vi "Find Nearest Neighbors Index Int.vi"(7 "#Neighbors":i32=1, 8 "error in (no error)":errorcluster, 10 "Points":i32[][](array[numeric]), 11 "KD Tree Int out":refnum<class "KD Tree Int.lvclass">) -> (0 "error out":errorcluster, 1 "Dists":sgl[][](array[numeric]), 2 "Indices":i32[][](array[numeric]), 3 "KD Tree Int out":refnum<class "KD Tree Int.lvclass">)   [LabVIEW 2020, in "KD Tree.lvlib" / "KD Tree Int.lvclass"]
uses:
  KD Tree Int.lvclass
  E:/Labview/LV 2020/Libs/flann/Classes/KD Tree/KD Tree.lvclass
  KD Tree/KD Tree.lvclass/KD Tree.ctl
  KD Tree/Read index_ptr.vi
  KD Tree/Read flann_params.vi
  KD Tree/Read Overwrite Lib Path.vi
  KD Tree.lvlib
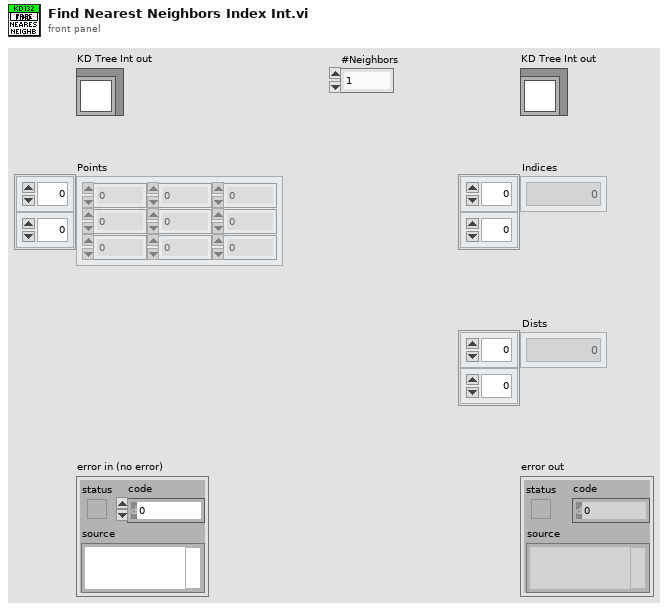
[diagram p1: front panel]
types:
  T1 = typedef "flann.lvlib/Flann Params.ctl" = cluster{"algorithm":u32, "checks":i32, "eps":sgl, "sorted":i32, "max_neighbors":i32, "cores":i32, "trees":i32, "leaf_max_size":i32, "branching":i32, "iterations":i32, "centers_init":u32, "cb_index":sgl, "target_precision":sgl, "build_weight":sgl, "memory_weight":sgl, "sample_fraction":sgl, "table_number_":u32, "key_size_":u32, "multi_probe_level_":u32, "log_level":u32, "random_seed":i32}
  T2 = typedef "KD Tree.lvlib/Flann Params.ctl" = cluster{"algorithm":u32, "checks":i32, "eps":sgl, "sorted":i32, "max_neighbors":i32, "cores":i32, "trees":i32, "leaf_max_size":i32, "branching":i32, "iterations":i32, "centers_init":u32, "cb_index":sgl, "target_precision":sgl, "build_weight":sgl, "memory_weight":sgl, "sample_fraction":sgl, "table_number_":u32, "key_size_":u32, "multi_probe_level_":u32, "log_level":u32, "random_seed":i32}
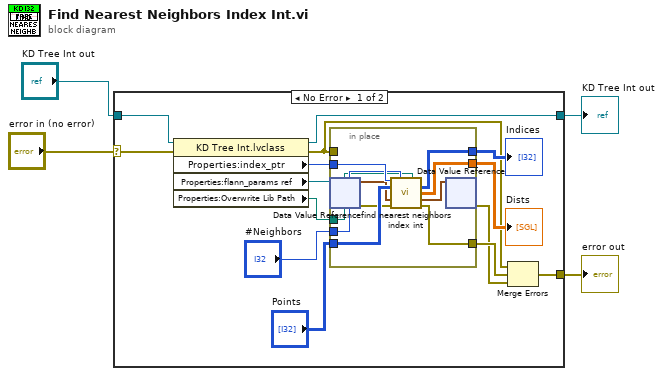
[diagram p0: block diagram]
diagram:
  n1 = case shown="No Error" "error in (no error)" {
    selector: "error in (no error)" -> [w18 w30]
    tunnel: [w9 w30] -> w3
    tunnel: [w16 w29] -> w1
    tunnel: "KD Tree Int out" -> [w17 w29]
    frame No Error {
      n2 = property class="KD Tree Int.lvclass"(reference=w17, error in=w18) -> (reference out=w16:refnum<class "KD Tree Int.lvclass">, error out=w5:errorcluster, "Properties:index_ptr"=w15:u64, "Properties:flann_params ref"=w12:refnum<data-value>, "Properties:Overwrite Lib Path"=w6:path)
      n3 = in-place {
        in-place-border: w15 -> [w28]
        in-place-border: "#Neighbors" -> [w27]
        in-place-border: "Points" -> [w26]
        in-place-border: [w22] -> w11
        in-place-border: [w21] -> w10
        in-place-border: [w20] -> w8
        in-place-border: w6 -> [w19]
        in-place-border: w5 -> [_]
        n4 = in-place-dvr #1(w12) -> (w25:T1, w24:errorcluster)
        n5 = call "find nearest neighbors index int.vi"("index_id"=w28, "nn"=w27, "Overwrite Lib Path"=w19, "testset"=w26, "flann_params"=w25, "error in (no error)"=w24) -> ("Indices"=w22:i32[][], "Dists"=w21:sgl[][], "flann_params"=w23:T2, "error out"=w20:errorcluster)  [unwired: 5 in, 1 out]
        n6 = in-place-dvr #1(w23) -> (w7:errorcluster)  [unwired: 1 out]
      }
      "Indices" <- w11
      "Dists" <- w10
      n7 = Merge Errors(w5, w8, w7) -> (w9:errorcluster)
    }
    frame Error {
    }
  }
  "error out" <- w3
  "KD Tree Int out" <- w1
